vi "RunningAverage.vi"() -> ()   [LabVIEW 2014]
panel:
  in  "정지":bool
  out "웨이브폼 차트":cluster{dbl, dbl}(graph)
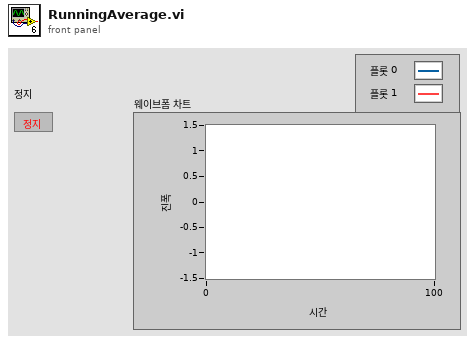
[diagram p1: front panel]
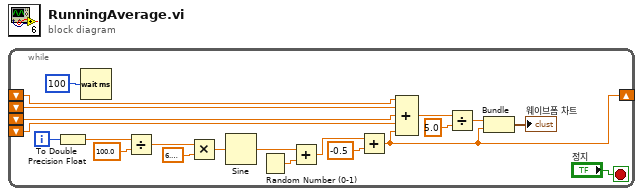
[diagram p0: block diagram]
diagram:
  n1 = while {
    shift-right: [w2] -> _
    shift-left: _ -> [w9]
    shift-left: _ -> [w8]
    shift-left: _ -> [w7]
    shift-left: _ -> [w6]
    i -> [w21]
    stop <- "정지" stop-if-true
    n2 = To Double Precision Float(number=w21) -> (double precision float=w20:dbl)
    n3 = Wait (ms)(milliseconds to wait=u32 100 ("대기 시간(ms)")) -> ()  [unwired: 1 out]
    n4 = Divide(x=w20, y=100.0) -> (x/y=w18:dbl)
    n5 = Multiply(x=w18, y=6.283185307179586) -> (x*y=w16:dbl)
    n6 = Sine(x=w16) -> (sin(x)=w15:dbl)
    n7 = Random Number (0-1)() -> (number: 0 to 1=w14:dbl)
    n8 = Add(x=w15, y=w14) -> (x+y=w13:dbl)
    n9 = Add(x=w13, y=-0.5) -> (x+y=w2:dbl)
    n10 = Compound Arithmetic op=ADD(w9, w8, w7, w6, w2) -> (w5:dbl)
    n11 = Divide(x=w5, y=5.0) -> (x/y=w3:dbl)
    n12 = Bundle(w3, w2) -> (→"웨이브폼 차트":cluster{dbl, dbl})  [unwired: 1 in]
  }
